vi "CD Read Engine_Parse Message_Update Channels Broadcast.vi"(8 "error in (no error)":errorcluster, 9 "NORESP":bool, 10 "Frame Descriptor":T2 {"RTs"."Status Channel Ref" format="%.0x"; "RTs"."Words Block Data Refs"."Data Reference" format="%.0x"; "RTs"."Timestamp Channel Data Reference" format="%.0x"; "BC"."Status Channel Refs" format="%.0x"; "BC"."Words Block Data Refs"."Data Reference" format="%.0x"; "BC"."Timestamp Channel Data Reference" format="%.0x"}, 11 "record in":T1 {"type" format="%04x"; "activity" format="%04x"; "error" format="%04x"; "cwd1" format="%04x"; "cwd2" format="%04x"; "swd1" format="%04x"; "swd2" format="%04x"; "data" format="%04x"}) -> (0 "error out":errorcluster, 3 "Timestamp (s)":dbl)   [LabVIEW 2017, in "Ballard MIL-1553 Engine.lvlib"]
uses:
  Ballard MIL-1553 Engine.lvlib
  Controls/RT Inline Broadcast Frame Descriptor.ctl
  Controls/RT Inline Frame Descriptor_BC.ctl
  <vilib>/NI Veristand/Custom Device API/Data Reference.ctl
  <vilib>/NI Veristand/Custom Device API/Block Data Reference.ctl
  <vilib>/NI Veristand/Custom Device API/Custom Device Item Ref.ctl
  Shared/Controls and Global/RT CWD2.ctl
  Shared/Controls and Global/RT CWD1.ctl
  Shared/Controls and Global/RT messageType.ctl
  Controls/RT Inline Frame Descriptor_RT.ctl
  <instrlib>/BTICardLib/Public/Controls/1553 Record.ctl
  <vilib>/NI Veristand/Custom Device API/Global Data Refs.vi
  <vilib>/NI VeriStand/Custom Device API/Custom Device API.lvlib
  Shared/Ballard 1553 Shared.lvlib
  <vilib>/NI VeriStand/Custom Device Tools/Custom Device Utility Library/Custom Device Utility Library.lvlib
  <instrlib>/BTICardLib/BTICardLV.lvlib
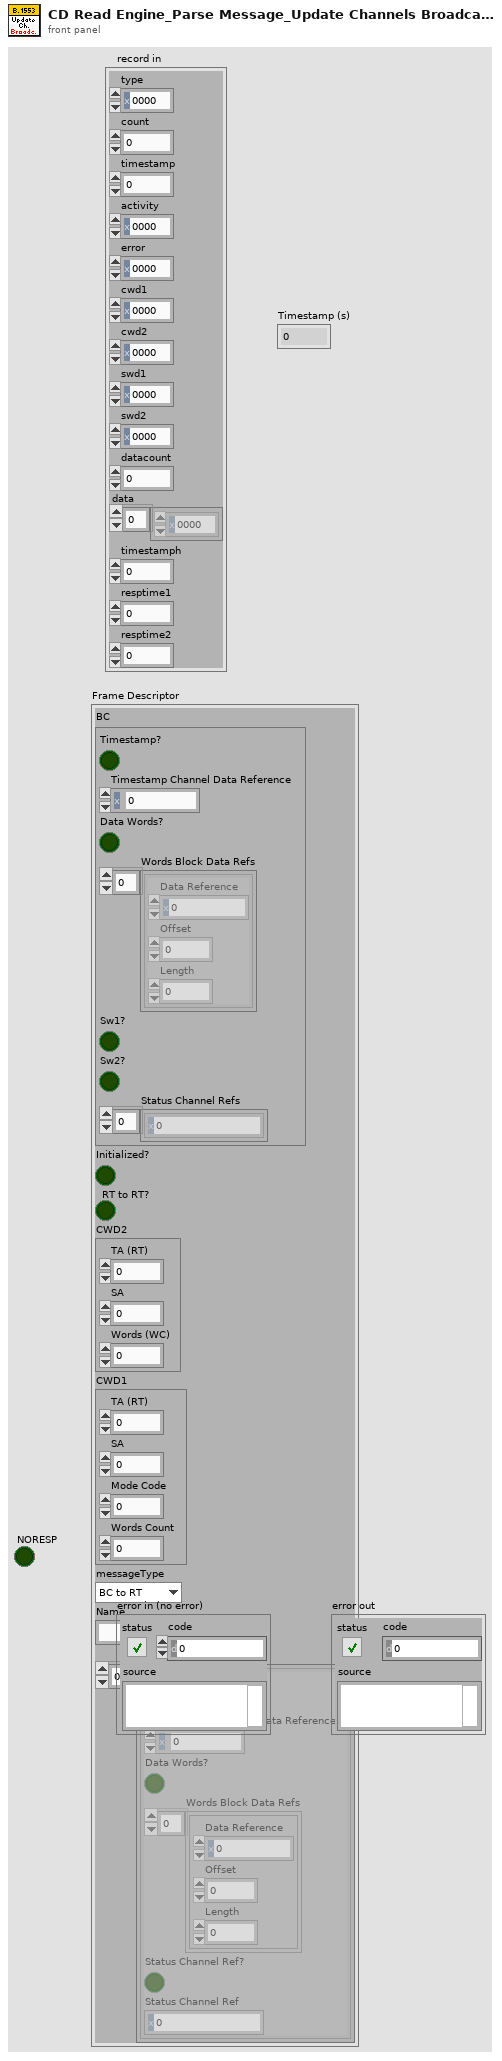
[diagram p1: front panel]
types:
  T1 = typedef "BTICardLV.lvlib/1553 Record.ctl" = cluster{"type":u16, "count":u16, "timestamp":u32, "activity":u16, "error":u16, "cwd1":u16, "cwd2":u16, "swd1":u16, "swd2":u16, "datacount":u16, "data":u16[], "timestamph":u32, "resptime1":u16, "resptime2":u16}
  T2 = typedef "Ballard MIL-1553 Engine.lvlib/RT Inline Broadcast Frame Descriptor.ctl" = cluster{"BC":T3, "Initialized?":bool, "RT to RT?":bool, "CWD2":T7, "CWD1":T8, "messageType":T9, "Name":string, "RTs":T10[]}
  T3 = typedef "Ballard MIL-1553 Engine.lvlib/RT Inline Frame Descriptor_BC.ctl" = cluster{"Timestamp?":bool, "Timestamp Channel Data Reference":T4, "Data Words?":bool, "Words Block Data Refs":T5[], "Sw1?":bool, "Sw2?":bool, "Status Channel Refs":T6[]}
  T4 = typedef "Custom Device API.lvlib/Data Reference.ctl" = i32
  T5 = typedef "Custom Device API.lvlib/Block Data Reference.ctl" = cluster{"Data Reference":T4, "Offset":u64, "Length":u64}
  T6 = typedef "Custom Device API.lvlib/Custom Device Item Ref.ctl" = u64
  T7 = typedef "Ballard 1553 Shared.lvlib/RT CWD2.ctl" = cluster{"TA (RT)":i8, "SA":i8, "Words (WC)":i8}
  T8 = typedef "Ballard 1553 Shared.lvlib/RT CWD1.ctl" = cluster{"TA (RT)":i8, "SA":i8, "Mode Code":i8, "Words Count":i8}
  T9 = typedef "Ballard 1553 Shared.lvlib/RT messageType.ctl" = enum16{"BC to RT", "RT to BC", "RT to RT", "MC (Rx)", "MC (Tx)"}
  T10 = typedef "Ballard MIL-1553 Engine.lvlib/RT Inline Frame Descriptor_RT.ctl" = cluster{"Timestamp?":bool, "Timestamp Channel Data Reference":T4, "Data Words?":bool, "Words Block Data Refs":T5[], "Status Channel Ref?":bool, "Status Channel Ref":T6}
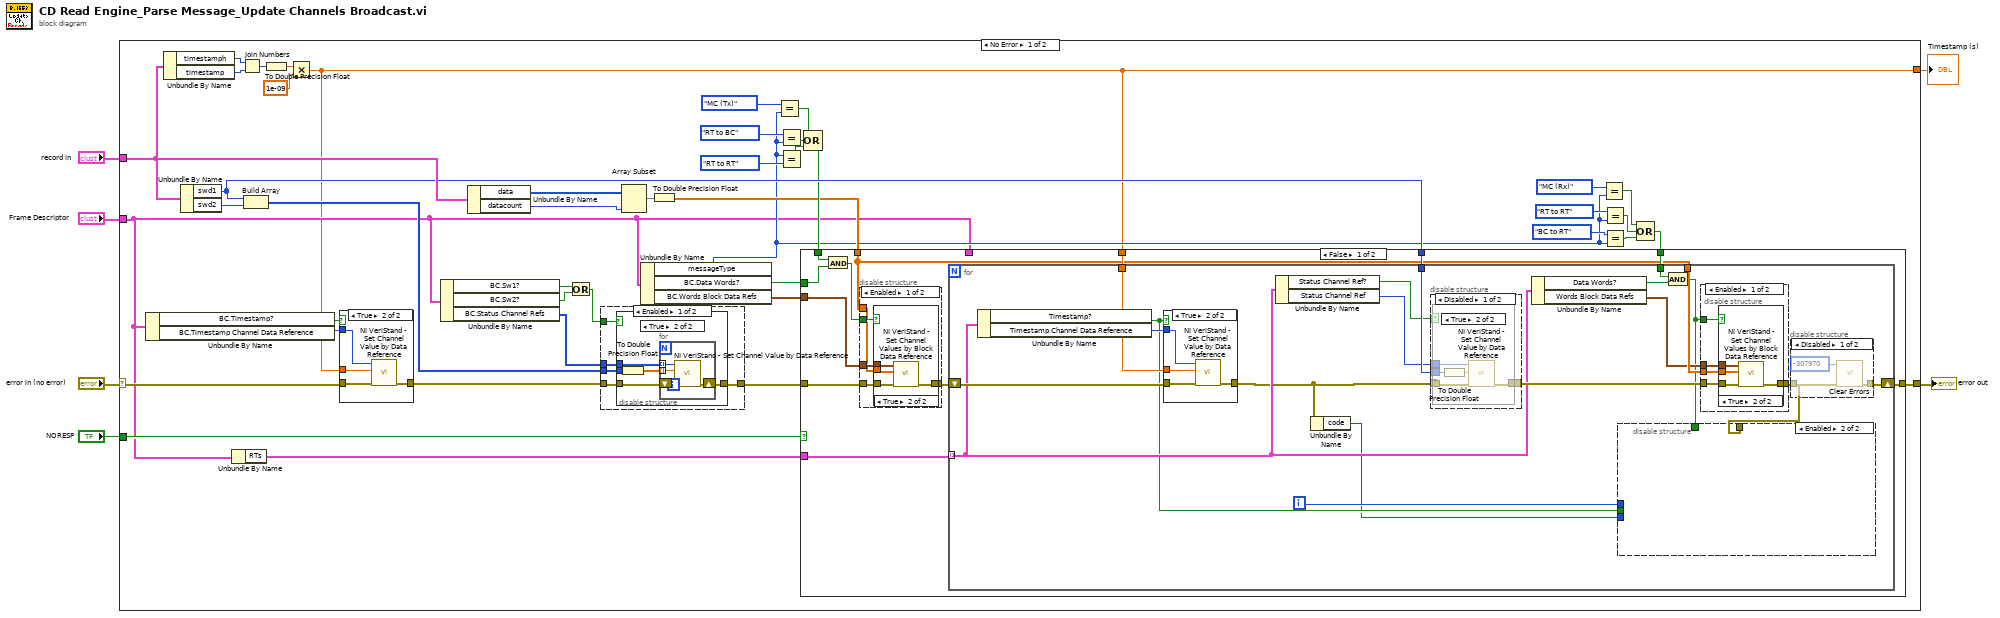
[diagram p0: block diagram]
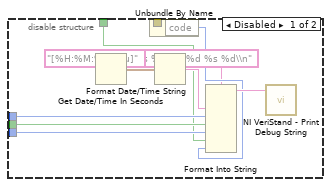
[diagram p2: hidden frame]
diagram:
  n1 = case shown="No Error" "error in (no error)" {
    selector: "error in (no error)" -> [w43 w158]
    tunnel: "Frame Descriptor" -> [w8 _]
    tunnel: [w38 w158] -> w5
    tunnel: "record in" -> [w39 _]
    tunnel: "NORESP" -> [w16 _]
    tunnel: [w7 _] -> w1
    frame No Error {
      n2 = Unbundle By Name(w8) -> ("BC.Timestamp?"=w45:bool, "BC.Timestamp Channel Data Reference"=w44:T4)
      n3 = Unbundle By Name(w39) -> ("timestamph"=w46:u32, "timestamp"=w47:u32)
      n4 = Unbundle By Name(w39) -> ("swd1"=w37:u16, "swd2"=w41:u16)
      n5 = Unbundle By Name(w8) -> ("RTs"=w9:T10[])
      n6 = Join Numbers(hi=w46, lo=w47) -> ((hi.lo)=w48:u64)
      n7 = Build Array(w37, w41) -> (w40:u16[])
      n8 = To Double Precision Float(number=w48) -> (double precision float=w49:dbl)
      n9 = Multiply(x=w49, y=1e-09) -> (x*y=w7:dbl)
      n10 = case shown="True" w45 {
        tunnel: w44 -> [_ w157]
        tunnel: w7 -> [_ w156]
        tunnel: w43 -> [w153 w155]
        tunnel: [w153 w154] -> w42
        frame False {
        }
        frame True {
          n11 = call <vilib>:"NI VeriStand - Set Channel Value by Data Reference.vi"("error in (no error)"=w155, "Value"=w156, "Data Reference in"=w157) -> ("error out"=w154:errorcluster)  [unwired: 8 in]
        }
      }
      n12 = Unbundle By Name(w8) -> ("BC.Sw1?"=w35:bool, "BC.Sw2?"=w36:bool, "BC.Status Channel Refs"=w33:T6[])
      n13 = Unbundle By Name(w39) -> ("data"=w30:u16[], "datacount"=w17:u16)
      n14 = Or(x=w35, y=w36) -> (x .or. y?=w34:bool)
      n15 = disable-structure shown="Enabled" {
        disable-tunnel: w42 -> [w141 w152]
        disable-tunnel: w40 -> [w140 _]
        disable-tunnel: w34 -> [w139 _]
        disable-tunnel: w33 -> [w138 _]
        disable-tunnel: [w137 w152] -> w32
        frame Enabled {
          n16 = case shown="True" w139 {
            tunnel: w138 -> [_ w147]
            tunnel: w140 -> [_ w146]
            tunnel: w141 -> [w142 w145]
            tunnel: [w142 w144] -> w137
            frame False {
            }
            frame True {
              n17 = To Double Precision Float(number=w146) -> (double precision float=w143:dbl[])
              n18 = for {
                tunnel: w147 -> [w151] mode=indexing
                tunnel: w143 -> [w150] mode=indexing
                shift-right: [w148] -> w144
                shift-left: w145 -> [w149]
                n19 = call <vilib>:"NI VeriStand - Set Channel Value by Data Reference.vi"("error in (no error)"=w149, "Value"=w150, "Data Reference in"=w151) -> ("error out"=w148:errorcluster)  [unwired: 8 in]
              }
            }
          }
        }
        frame Disabled {
        }
      }
      n20 = Array Subset(array=w30, length=w17) -> (w29:u16[])  [unwired: 1 in]
      n21 = Unbundle By Name(w8) -> ("messageType"=w10:T9, "BC.Data Words?"=w21:bool, "BC.Words Block Data Refs"=w31:T5[])
      n22 = To Double Precision Float(number=w29) -> (double precision float=w18:dbl[])
      n23 = Equal?(x=RT_messageType."MC (Tx)", y=w10) -> (x = y?=w11:bool)
      n24 = Equal?(x=RT_messageType."RT to BC", y=w10) -> (x = y?=w23:bool)
      n25 = Equal?(x=w10, y=RT_messageType."RT to RT") -> (x = y?=w22:bool)
      n26 = Compound Arithmetic op=OR(w11, w23, w22) -> (w27:bool)
      n27 = Equal?(x=RT_messageType."MC (Rx)", y=w10) -> (x = y?=w13:bool)
      n28 = Equal?(x=RT_messageType."RT to RT", y=w10) -> (x = y?=w20:bool)
      n29 = Equal?(x=RT_messageType."BC to RT", y=w10) -> (x = y?=w19:bool)
      n30 = Compound Arithmetic op=OR(w13, w20, w19) -> (w25:bool)
      n31 = case shown="False" w16 {
        tunnel: w7 -> [w62 _]
        tunnel: [w61 w136] -> w38
        tunnel: w8 -> [_ _]
        tunnel: w37 -> [w60 _]
        tunnel: w32 -> [w59 w136]
        tunnel: w31 -> [w58 _]
        tunnel: w27 -> [w55 _]
        tunnel: w25 -> [w54 _]
        tunnel: w21 -> [w53 _]
        tunnel: w18 -> [w52 _]
        tunnel: w9 -> [w51 _]
        frame False {
          n32 = And(x=w55, y=w53) -> (x .and. y?=w56:bool)
          n33 = disable-structure shown="Enabled" {
            disable-tunnel: w56 -> [w129 _]
            disable-tunnel: w59 -> [w128 w135]
            disable-tunnel: w58 -> [w127 _]
            disable-tunnel: [w126 w135] -> w57
            disable-tunnel: w52 -> [w125 _]
            frame Enabled {
              n34 = case shown="True" w129 {
                tunnel: w128 -> [w130 w134]
                tunnel: w127 -> [_ w133]
                tunnel: w125 -> [_ w132]
                tunnel: [w130 w131] -> w126
                frame False {
                }
                frame True {
                  n35 = call <vilib>:"NI VeriStand - Set Channel Values by Block Data Reference.vi"("error in (no error)"=w134, "Values Array in"=w132, "Block Data Ref"=w133) -> ("error out"=w131:errorcluster)  [unwired: 6 in, 2 out]
                }
              }
            }
            frame Disabled {
            }
          }
          n36 = for {
            tunnel: w62 -> [w81]
            tunnel: w60 -> [w80]
            tunnel: w54 -> [w77]
            tunnel: w52 -> [w76]
            tunnel: w51 -> [w70] mode=indexing
            shift-right: [w69] -> w61
            shift-left: w57 -> [w78]
            i -> [w68]
            n37 = Unbundle By Name(w70) -> ("Timestamp?"=w67:bool, "Timestamp Channel Data Reference"=w79:T4)
            n38 = case shown="True" w67 {
              tunnel: w79 -> [_ w124]
              tunnel: w81 -> [_ w123]
              tunnel: w78 -> [w120 w122]
              tunnel: [w120 w121] -> w66
              frame False {
              }
              frame True {
                n39 = call <vilib>:"NI VeriStand - Set Channel Value by Data Reference.vi"("error in (no error)"=w122, "Value"=w123, "Data Reference in"=w124) -> ("error out"=w121:errorcluster)  [unwired: 8 in]
              }
            }
            n40 = Unbundle By Name(w70) -> ("Status Channel Ref?"=w73:bool, "Status Channel Ref"=w74:T6)
            n41 = Unbundle By Name(w66) -> ("code"=w65:i32)
            n42 = disable-structure shown="Disabled" {
              disable-tunnel: w80 -> [w112 _]
              disable-tunnel: w74 -> [w111 _]
              disable-tunnel: w73 -> [w110 _]
              disable-tunnel: w66 -> [w109 w119]
              disable-tunnel: [w108 w119] -> w72
              frame Disabled {
                n43 = case shown="True" w110 {
                  tunnel: w111 -> [_ w116]
                  tunnel: [w113 w117] -> w108
                  tunnel: w109 -> [w113 w118]
                  tunnel: w112 -> [_ w115]
                  frame False {
                  }
                  frame True {
                    n44 = To Double Precision Float(number=w115) -> (double precision float=w114:dbl)
                    n45 = call <vilib>:"NI VeriStand - Set Channel Value by Data Reference.vi"("error in (no error)"=w118, "Value"=w114, "Data Reference in"=w116) -> ("error out"=w117:errorcluster)  [unwired: 8 in]
                  }
                }
              }
              frame Enabled {
              }
            }
            n46 = Unbundle By Name(w70) -> ("Data Words?"=w71:bool, "Words Block Data Refs"=w75:T5[])
            n47 = And(x=w77, y=w71) -> (x .and. y?=w63:bool)
            n48 = disable-structure shown="Enabled" {
              disable-tunnel: [w101 w107] -> w64
              disable-tunnel: w75 -> [w100 _]
              disable-tunnel: w63 -> [w99 _]
              disable-tunnel: w76 -> [w98 _]
              disable-tunnel: w72 -> [w97 w107]
              frame Enabled {
                n49 = case shown="True" w99 {
                  tunnel: w97 -> [w102 w106]
                  tunnel: w100 -> [_ w105]
                  tunnel: [w102 w104] -> w101
                  tunnel: w98 -> [_ w103]
                  frame False {
                  }
                  frame True {
                    n50 = call <vilib>:"NI VeriStand - Set Channel Values by Block Data Reference.vi"("error in (no error)"=w106, "Values Array in"=w103, "Block Data Ref"=w105) -> ("error out"=w104:errorcluster)  [unwired: 6 in, 2 out]
                  }
                }
              }
              frame Disabled {
              }
            }
            n51 = disable-structure shown="Enabled" {
              disable-tunnel: w68 -> [w88 _]
              disable-tunnel: w67 -> [w87 _]
              disable-tunnel: w65 -> [w86 _]
              disable-tunnel: w64 -> [w85 _]
              disable-tunnel: w63 -> [w84 _]
              frame Disabled {
                n52 = Get Date/Time In Seconds() -> (seconds since 1Jan1904=w91:timestamp)
                n53 = Unbundle By Name(w85) -> ("code"=w83:i32)
                n54 = Format Date/Time String(time format string (%c)="[%H:%M:%S%3u]", seconds (now)=w91) -> (date/time string=w89:string)  [unwired: 1 in]
                n55 = Format Into String(format string="%s %d %s %d %s %d\\n", w89, w88, w87, w86, w84, w83) -> (resulting string=w92:string)  [unwired: 2 in, 1 out]
                n56 = call <vilib>:"NI VeriStand - Print Debug String.vi"("Message"=w92) -> ()  [unwired: 10 in, 1 out]
              }
              frame Enabled {
              }
            }
            n57 = disable-structure shown="Disabled" {
              disable-tunnel: [w95 w96] -> w69
              disable-tunnel: w64 -> [w93 w96]
              frame Disabled {
                n58 = call <vilib>:"Clear Errors.vi"("error in (no error)"=w93, "specific error code to clear (0: all)"=-307970) -> ("error out"=w95:errorcluster)  [unwired: 4 in, 1 out]
              }
              frame Enabled {
              }
            }
          }
        }
        frame True {
          # "NO RESPONSE from RT."
        }
      }
    }
    frame Error {
    }
  }
  "error out" <- w5
  "Timestamp (s)" <- w1
